vi "StimFile-Initialize.vi"(0 "File":T1, 7 "Npts":i32=-1, 11 "error in (no error)":errorcluster) -> (4 "File out":T1, 15 "error out":errorcluster)   [LabVIEW 2020]
uses:
  StimFile-Params.ctl
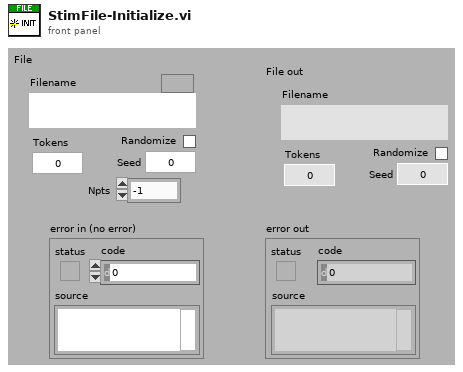
[diagram p1: front panel]
types:
  T1 = typedef "StimFile-Params.ctl" = cluster{"Filename":path, "Signal":dbl[], "Channel":i32, "stream":bool, "offset":i32, "nreps":i32, "loops":i32, "Randomize":bool, "order":i32[], "Seed":i32, "Tokens":i32}
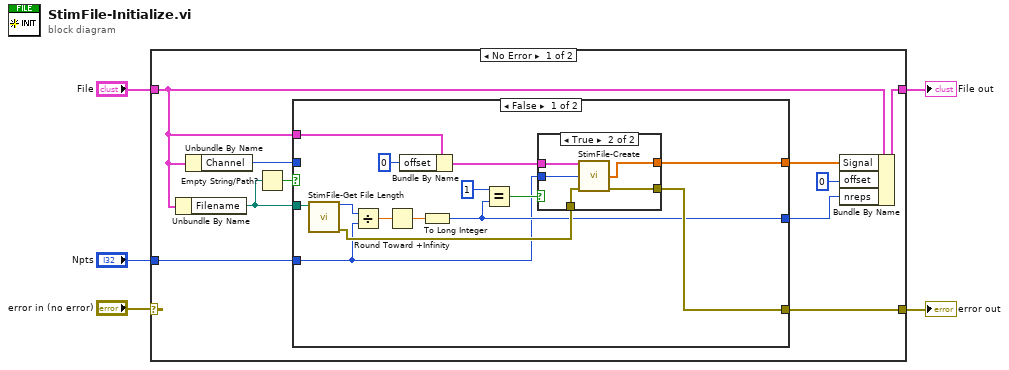
[diagram p0: block diagram]
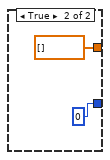
[diagram p3: hidden frame]
diagram:
  n1 = case shown="No Error" "error in (no error)" {
    selector: "error in (no error)" -> [_ w38]
    tunnel: "File" -> [w6 _]
    tunnel: "Npts" -> [w13 _]
    tunnel: [w15 w38] -> w2
    tunnel: [w14 _] -> w1
    frame No Error {
      n2 = Unbundle By Name(w6) -> ("Filename"=w10:path)
      n3 = Unbundle By Name(w6) -> ("Channel"=w9:i32)
      n4 = Empty String/Path?(string/path=w10) -> (empty?=w11:bool)
      n5 = case shown="False" w11 {
        tunnel: w10 -> [w29 _]
        tunnel: [w18 _] -> w15
        tunnel: w13 -> [w16 _]
        tunnel: [w20 dbl[] [] ("Y")] -> w12
        tunnel: w9 -> [_ _]
        tunnel: [w17 0] -> w7
        tunnel: w6 -> [w24 _]
        frame False {
          n6 = call "StimFile-Get File Length.vi"("Filename"=w29) -> ("total number of samples/ch"=w28:u32, "error out"=w19:errorcluster)  [unwired: 13 in]
          n7 = Divide(x=w28, y=w16) -> (x/y=w27:dbl)
          n8 = Round Toward +Infinity(x=w27) -> (ceil(x): smallest int >= x=w26:dbl)
          n9 = Bundle By Name(cluster=w24, "offset"=0) -> (w22:T1)
          n10 = To Long Integer(number=w26) -> (32bit integer=w17:i32)
          n11 = Equal?(x=1, y=w17) -> (x = y?=w21:bool)
          n12 = case shown="True" w21 {
            tunnel: w22 -> [_ w35]
            tunnel: [_ w34] -> w20
            tunnel: w19 -> [w30 w33]
            tunnel: [w30 w32] -> w18
            tunnel: w16 -> [_ w31]
            frame False {
            }
            frame True {
              n13 = call "StimFile-Create.vi"("File"=w35, "Npts"=w31, "error in (no error)"=w33) -> ("Y"=w34:dbl[], "error out"=w32:errorcluster)  [unwired: 10 in, 1 out]
            }
          }
        }
        frame True {
        }
      }
      n14 = Bundle By Name(cluster=w6, "Signal"=w12, "offset"=0, "nreps"=w7) -> (w14:T1)
    }
    frame Error {
    }
  }
  "error out" <- w2
  "File out" <- w1
